vi "NI 9213 Getting Started (FPGA).vi"() -> ()   [LabVIEW 2011]
doc: "This VI continually reads single point values from all four channels of the NI 9211."
uses:
  <vilib>/LabVIEW Targets/FPGA/cRIO/shared/nicrio_ModuleControls/nicrio_BasicConversionTime.ctl
  <vilib>/rvi/eio/common/nirviEmuTemplatePropertySet_errors.vi
  <vilib>/rvi/eio/common/nirviEmuTemplateMethod_errors.vi
  <vilib>/eio/EIOPropertyNode/EIOPropertyNode.xnode
  <vilib>/eio/EIONode/EIONode.xnode
  <vilib>/eio/EIOMethodNode/EIOMethodNode.xnode
  <vilib>/rvi/eio/common/nirviEmuTemplatePropertyGet_errors.vi
  <vilib>/rvi/eio/common/nirviEmuTemplatePropertyGet_noerrors.vi
  <vilib>/rvi/eio/common/nirviEmuTemplatePropertySet_noerrors.vi
panel:
  out "TC Status":T1
  out "FPGA Error Out":errorcluster
  out "TC Output":T2 {"Mod1/TC0" format="%.26g"; "Mod1/TC1" format="%.26g"; "Mod1/TC2" format="%.26g"; "Mod1/TC3" format="%.26g"; "Mod1/TC4" format="%.26g"; "Mod1/TC5" format="%.26g"; "Mod1/TC6" format="%.26g"; "Mod1/TC7" format="%.26g"; "Mod1/TC8" format="%.26g"; "Mod1/TC9" format="%.26g"; "Mod1/TC10" format="%.26g"; "Mod1/TC11" format="%.26g"; "Mod1/TC12" format="%.26g"; "Mod1/TC13" format="%.26g"; "Mod1/TC14" format="%.26g"; "Mod1/TC15" format="%.26g"; "Mod1/AutoZero" format="%.26g"; "Mod1/CJC" format="%.26g"}
  in  "Conversion Time":T3=enum."High Resolution"
  in  "Update Conversion Time":bool
  in  "Stop":bool
  # "For instructions, and select Help>>Show Context Help and hover over the icon."
  # "TC Status"
  # "TC Outputs"
  # "Input Parameters"
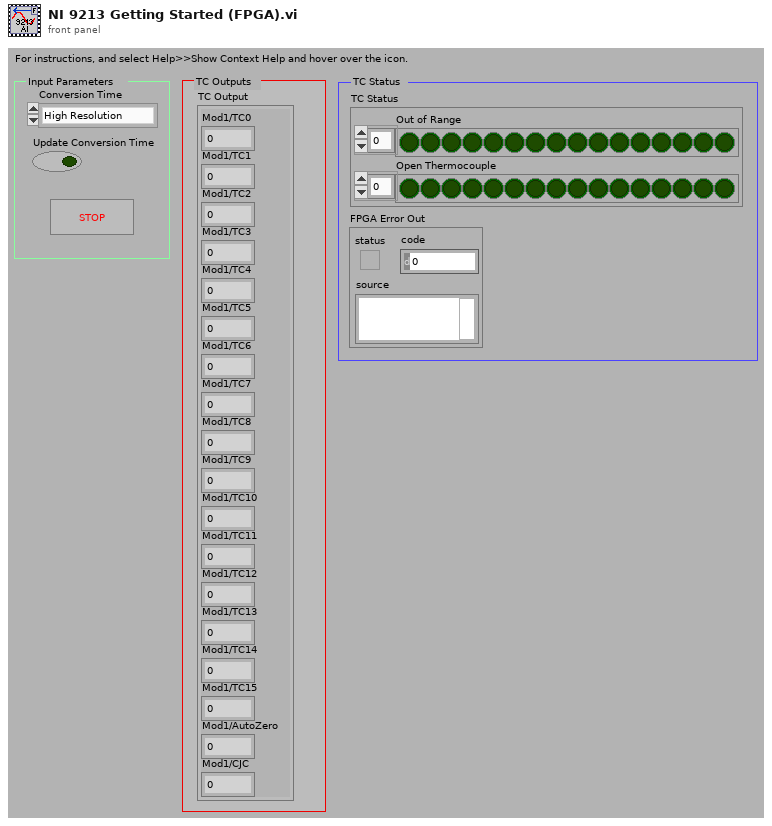
[diagram p1: front panel]
types:
  T1 = cluster{"Out of Range":bool[], "Open Thermocouple":bool[]}
  T2 = cluster{"Mod1/TC0":fxp<+/-,24,-2>, "Mod1/TC1":fxp<+/-,24,-2>, "Mod1/TC2":fxp<+/-,24,-2>, "Mod1/TC3":fxp<+/-,24,-2>, "Mod1/TC4":fxp<+/-,24,-2>, "Mod1/TC5":fxp<+/-,24,-2>, "Mod1/TC6":fxp<+/-,24,-2>, "Mod1/TC7":fxp<+/-,24,-2>, "Mod1/TC8":fxp<+/-,24,-2>, "Mod1/TC9":fxp<+/-,24,-2>, "Mod1/TC10":fxp<+/-,24,-2>, "Mod1/TC11":fxp<+/-,24,-2>, "Mod1/TC12":fxp<+/-,24,-2>, "Mod1/TC13":fxp<+/-,24,-2>, "Mod1/TC14":fxp<+/-,24,-2>, "Mod1/TC15":fxp<+/-,24,-2>, "Mod1/AutoZero":fxp<+/-,24,-2>, "Mod1/CJC":fxp<+/-,24,-2>}
  T3 = typedef "nicrio_BasicConversionTime.ctl" = enum8{"High Speed", "High Resolution"}
  T4 = cluster{"TC1X":fxp<+/-,24,-2>, "TC2A":fxp<+/-,24,-2>, "TC3Y":fxp<+/-,24,-2>, "TC4B":fxp<+/-,24,-2>, "TC5":fxp<+/-,24,-2>, "TC6":fxp<+/-,24,-2>, "TC7":fxp<+/-,24,-2>, "TC8":fxp<+/-,24,-2>, "TC9":fxp<+/-,24,-2>, "TC10":fxp<+/-,24,-2>, "TC11":fxp<+/-,24,-2>, "TC12":fxp<+/-,24,-2>, "TC13":fxp<+/-,24,-2>, "TC14":fxp<+/-,24,-2>, "TC15":fxp<+/-,24,-2>, "TC16":fxp<+/-,24,-2>, "Mod4/Autozero":fxp<+/-,24,-2>, "Mod4/CJC":fxp<+/-,24,-2>}
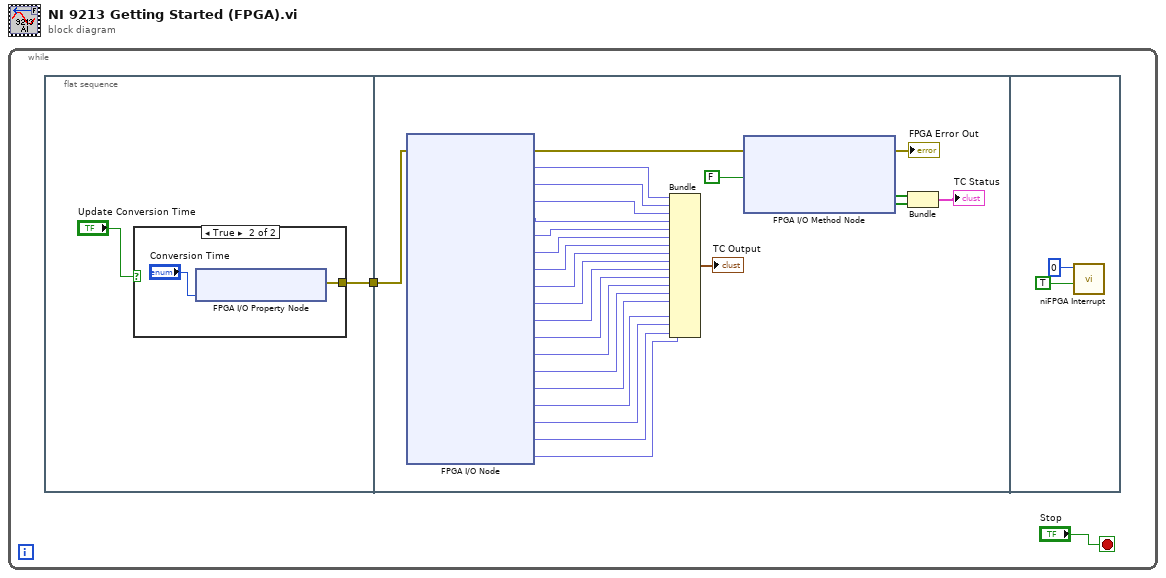
[diagram p0: block diagram]
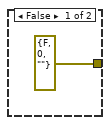
[diagram p2: hidden frame]
diagram:
  n1 = while {
    stop <- "Stop" stop-if-true
    n2 = flat-sequence {
      tunnel: [w3] -> w1
      tunnel: w1 -> [w25]
      frame #0 {
        n3 = case shown="True" "Update Conversion Time" {
          tunnel: [errorcluster {"status"=FALSE, "code"=0, "source"=""} ("error out") w6] -> w3
          frame False {
          }
          frame True {
            n4 = xnode "FPGA I/O Property Node"("Conversion Time"="Conversion Time") -> ("error out"=w6:errorcluster)  [unwired: 2 in, 1 out]
          }
        }
      }
      frame #1 {
        n5 = xnode "FPGA I/O Node"("error in"=w25) -> ("error out"=w31:errorcluster, "TC1X"=w33:fxp<+/-,24,-2>, "TC2A"=w24:fxp<+/-,24,-2>, "TC3Y"=w23:fxp<+/-,24,-2>, "TC4B"=w22:fxp<+/-,24,-2>, "TC5"=w21:fxp<+/-,24,-2>, "TC6"=w20:fxp<+/-,24,-2>, "TC7"=w19:fxp<+/-,24,-2>, "TC8"=w18:fxp<+/-,24,-2>, "TC9"=w17:fxp<+/-,24,-2>, "TC10"=w16:fxp<+/-,24,-2>, "TC11"=w15:fxp<+/-,24,-2>, "TC12"=w14:fxp<+/-,24,-2>, "TC13"=w13:fxp<+/-,24,-2>, "TC14"=w12:fxp<+/-,24,-2>, "TC15"=w11:fxp<+/-,24,-2>, "TC16"=w10:fxp<+/-,24,-2>, "Mod4/Autozero"=w9:fxp<+/-,24,-2>, "Mod4/CJC"=w8:fxp<+/-,24,-2>)  [unwired: 18 in, 18 out]
        n6 = Bundle("TC1X"=w33, "TC2A"=w24, "TC3Y"=w23, "TC4B"=w22, "TC5"=w21, "TC6"=w20, "TC7"=w19, "TC8"=w18, "TC9"=w17, "TC10"=w16, "TC11"=w15, "TC12"=w14, "TC13"=w13, "TC14"=w12, "TC15"=w11, "TC16"=w10, "Mod4/Autozero"=w9, "Mod4/CJC"=w8) -> (→"TC Output":T4)  [unwired: 1 out]
        n7 = xnode "FPGA I/O Method Node"("error in"=w31, "Force Status Read"=FALSE) -> ("error out"=→"FPGA Error Out":errorcluster, "Out Of Range"=w28:bool[], "Open"=w27:bool[])  [unwired: 1 in, 1 out]
        n8 = Bundle("Out Of Range"=w28, "Open"=w27) -> (→"TC Status":cluster{"Out Of Range":bool[], "Open":bool[]})  [unwired: 1 out]
      }
      frame #2 {
        n9 = call <vilib>:"niFPGA Interrupt.vi"("Wait Until Cleared"=TRUE, "IRQ Number"=u8 0 ("IRQ Bit (0-31)")) -> ()  [unwired: 1 in]
      }
    }
  }
